vi "Ball Align.vi"(11 "Robot Velocities In":T2) -> (3 "Robot Velocities Out":T2)   [LabVIEW 2025]
uses:
  <vilib>/Analysis/NI_AAL_Angle.lvlib
  <vilib>/Analysis/coordinate.llb/Wrap Angle (scalar).vi
  <vilib>/Analysis/coordinate.llb/Angle Units.ctl
  Framework/Robot Global Data.vi
  swerve-template/Type Definitions/Data/Robot Velocities.ctl
panel:
  in  "output range":cluster{"high":dbl, "low":dbl}={"high"=100.0, "low"=-100.0} {"low" format="%.2f"; "high" format="%.2f"}
  in  "advanced":cluster{"alpha":dbl, "i-zone":dbl}={"alpha"=nan, "i-zone"=nan} {"i-zone" format="%.2f"; "alpha" format="%.2f"}
  in  "PID gains":T1={"proportional gain (Kp)"=10.0, "integral time (Ki)"=0.0, "derivative time (Kd)"=0.0} {"derivative time (Kd)" format="%.3f"; "integral time (Ki)" format="%.3f"; "proportional gain (Kp)" format="%.3f"}
  out "Err/Out Chart":cluster{dbl, dbl}(graph)
  out "SP/PV Chart":cluster{"setpoint":dbl, "process variable":dbl}(graph)
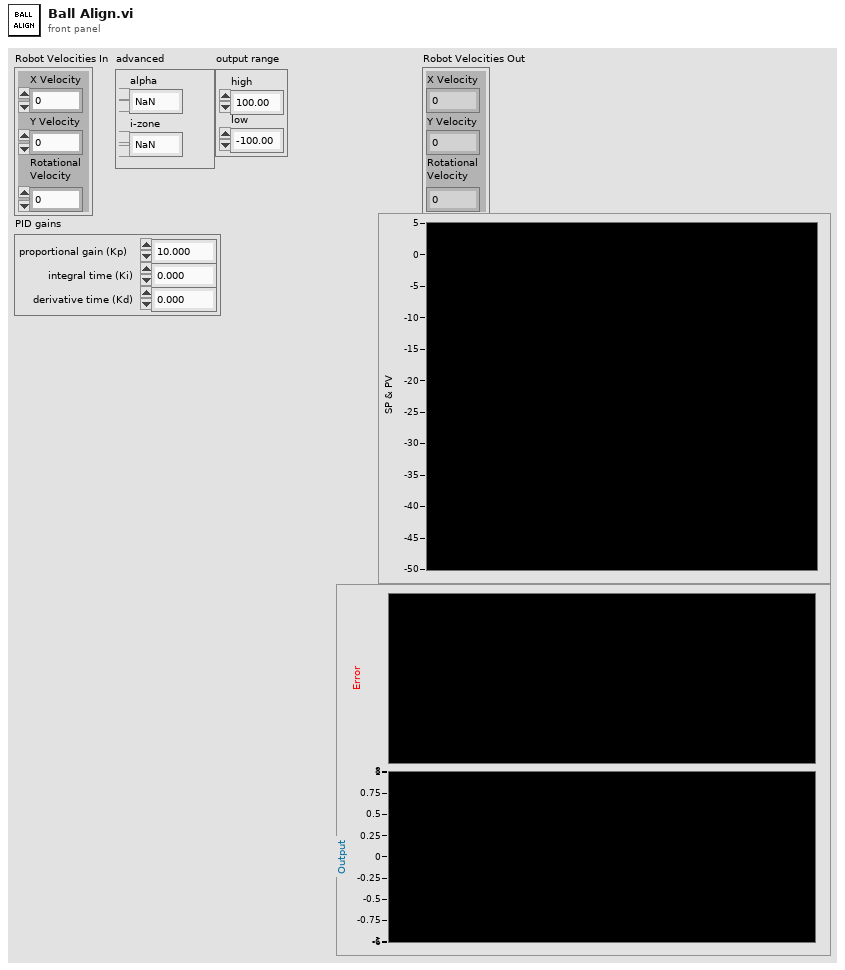
[diagram p1: front panel]
types:
  T1 = cluster{"proportional gain (Kp)":dbl, "integral time (Ki)":dbl, "derivative time (Kd)":dbl}
  T2 = typedef "Robot Velocities.ctl" = cluster{"X Velocity":dbl, "Y Velocity":dbl, "Rotational \nVelocity":dbl}
  T3 = typedef "NI_AAL_Angle.lvlib/Angle Units.ctl" = i32
  T4 = cluster{"Ball Direction":dbl, "Ball Distance":dbl}[]
  T5 = cluster{"Ball Direction":dbl, "Ball Distance":dbl}
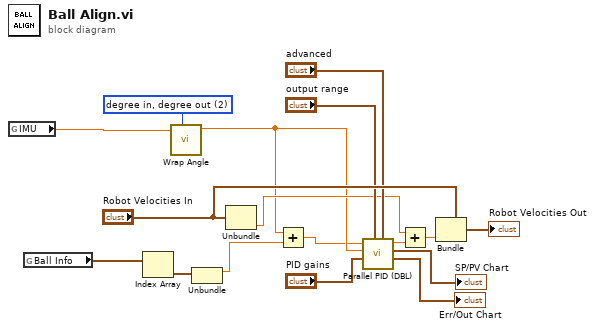
[diagram p0: block diagram]
diagram:
  w7 = T3 2 items=["radian in, radian out", "radian in, degree out", "degree in, degree out", "degree in, radian out"] ("angle units")
  n1 = global read "Robot Global Data.vi" "IMU"() -> (w6:dbl)
  n2 = global read "Robot Global Data.vi" "Ball Info"() -> (w5:T4)
  n3 = Index Array(array=w5) -> (element=w4:T5)  [unwired: 1 in]
  n4 = call-poly <vilib>:"Wrap Angle.vi"("angle units"=w7, "angle in"=w6) -> ("angle out"=w3:dbl)  [unwired: 8 in, 1 out]
  n5 = Unbundle(w4) -> ("Ball Direction"=w2:dbl)  [unwired: 1 out]
  n6 = Unbundle("Robot Velocities In") -> ("Rotational \nVelocity"=w9:dbl)  [unwired: 2 out]
  n7 = Add(x=w3, y=w2) -> (x+y=w1:dbl)
  n8 = call <vilib>:"Parallel PID (DBL).vi"("advanced"="advanced", "output range"="output range", "PID gains"="PID gains", "process variable"=w3, "setpoint"=w1) -> ("Err/Out Chart"=→"Err/Out Chart":cluster{dbl, dbl}, "SP/PV Chart"=→"SP/PV Chart":cluster{"setpoint":dbl, "process variable":dbl}, "output"=w10:dbl)  [unwired: 3 in, 1 out]
  n9 = Add(x=w9, y=w10) -> (x+y=w8:dbl)
  n10 = Bundle(cluster="Robot Velocities In", "Rotational \nVelocity"=w8) -> (→"Robot Velocities Out":T2)  [unwired: 2 in]
